vi "NMEA Example - serial.vi"() -> ()   [LabVIEW 2016, in "环境动力监测库.lvlib" / "AIRMAR WeatherCaster.lvlib"]
uses:
  AIRMAR WeatherCaster.lvlib
  NMEA_GPRMC-data.ctl
  NMEA_LatitudeDirection.ctl
  NMEA_LongitudeDirection.ctl
  NMEA_GPVTG-data.ctl
  NMEA_Mode.ctl
  NMEA_GPGGA-data.ctl
  NMEA_GPS-Quality.ctl
  <vilib>/Instr/_visa.llb/VISA Flush IO Buffer Mask.ctl
  <vilib>/Instr/_visa.llb/VISA Configure Serial Port (Instr).vi
panel:
  out "Longitude [deg]":string
  out "Latitude [deg]":string
  in  "time zone":i32
  out "Time":string
  in  "Stop":bool
  in  "VISA":refnum<visa-resource-name>
  in  "Data file path":path
  out "Data":string[][](table)
  out "Raw data GPS":string
  in  "Buffer Size":u32=6400
  in  "Baud rate":u32=115200
  out "TX LAT":dbl
  out "TX LONG":dbl
  out "$GPGGA-message_OUT":T1={"TimeStamp"=timestamp(0 s since 1904-01-01), "Latitude"=0.0, "Latitude-Direction"=enum."", "Longitude"=1.0, "Longitude-Direction"=enum."", "GPS-Quality"=enum."GPS fix (SPS)", "Number of Satellites"=0, "Horizontal Dilution of Precision"=0.0, "Altitude above Mean-Sea-Level"=0.0, "Geoidal separation"=0.0, "Time since last DGPS update"=0.0, "DGPS reference station ID"=0} {"Time since last DGPS update" format="%.02f [s]"; "Geoidal separation" format="%.02f [m]"; "Altitude above Mean-Sea-Level" format="%.02f [m]"; "Horizontal Dilution of Precision" format="%.02f [HDOP]"; "Longitude" format="%0.4f [long]"; "Latitude" format="%.04f [lat]"; "TimeStamp" format="%<%.2X>T"}
  out "$GPVTG-message_OUT":T5={"True Course over Ground"=0.0, "Magnetic Course over Ground"=0.0, "Speed over Ground in knots"=0.0, "Speed over Ground in km/h"=1.0, "Mode"=""} {"Speed over Ground in km/h" format="%.02f [km/h]"; "Speed over Ground in knots" format="%.02f [kts]"; "Magnetic Course over Ground" format="%.02f [deg]"; "True Course over Ground" format="%.02f [deg]"}
  out "$GPRMC-message_OUT":T7={"TimeStamp"=timestamp(0 s since 1904-01-01), "Validity"=FALSE, "Latitude"=0.0, "Latitude-Direction"=enum."North", "Longitude"=0.0, "Longitude-Direction"=enum."East", "Speed in knots"=0.0, "True course"=0.0, "Date Stamp"=timestamp(0 s since 1904-01-01), "Magnetic Variation (East/West)"=0.0} {"Magnetic Variation (East/West)" format="%.02f [deg]"; "Date Stamp" format="%<%x>T"; "True course" format="%.02f [deg]"; "Speed in knots" format="%.02f [kts]"; "Longitude" format="%0.4f [long]"; "Latitude" format="%.04f [lat]"; "TimeStamp" format="%<%.2X>T"}
  # "NMEA EXAMPLE WITH VISA SERIAL"
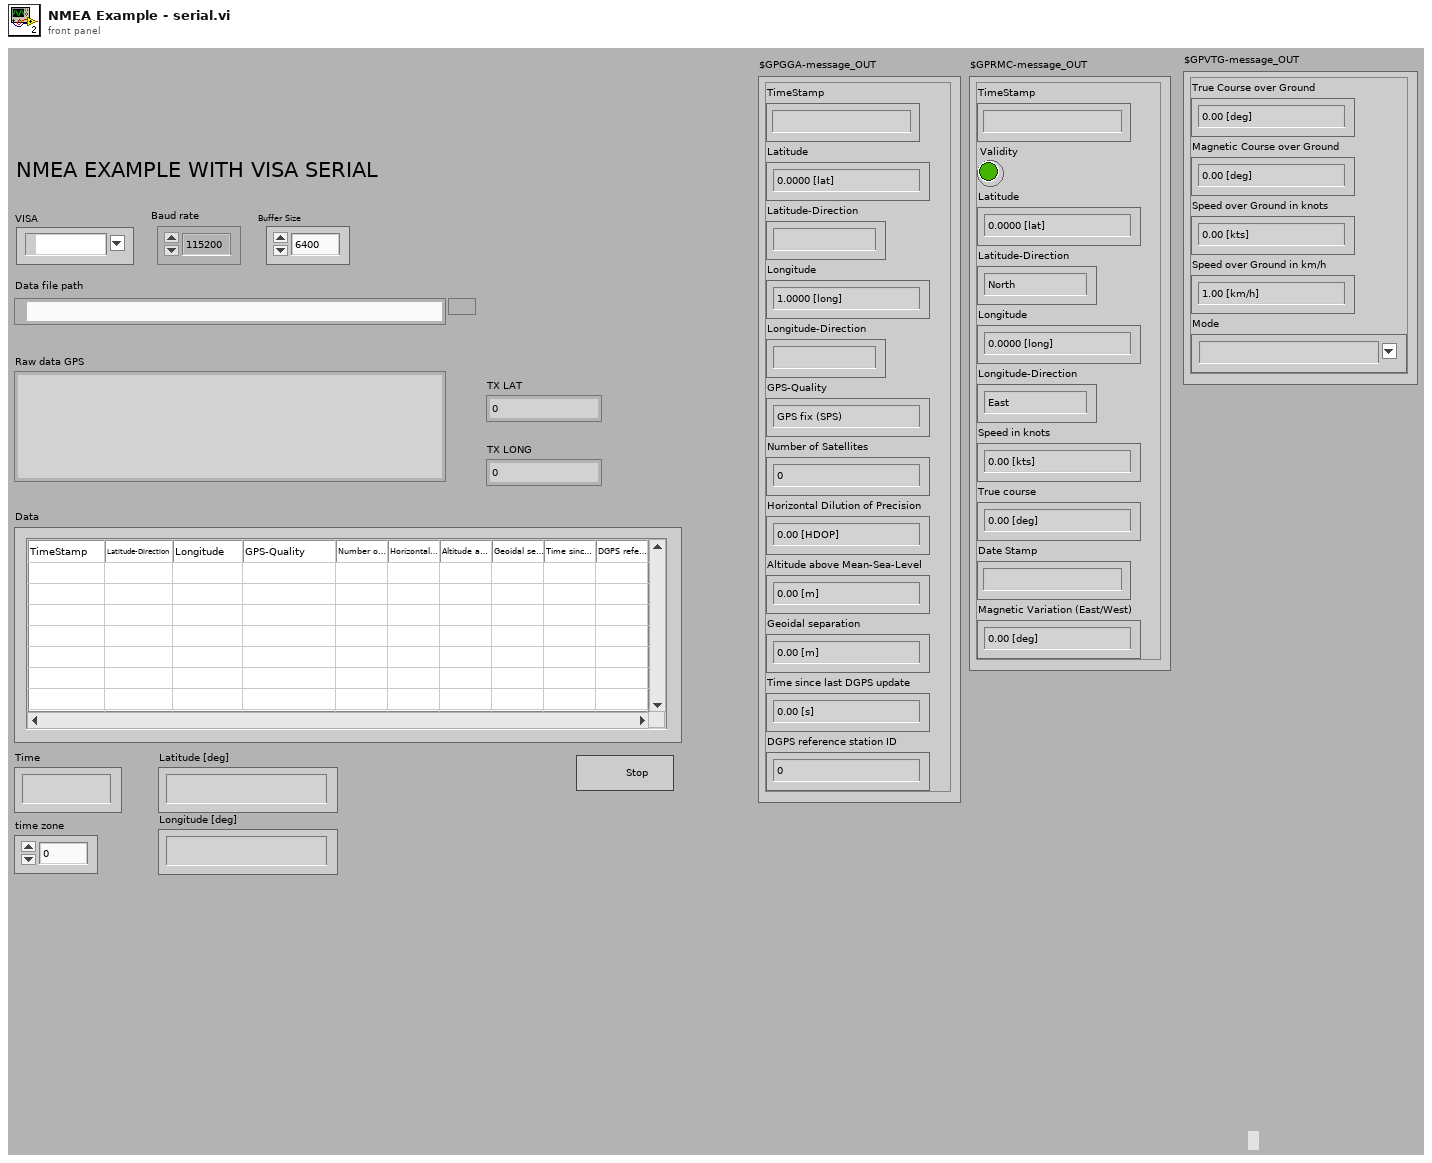
[diagram p1: front panel]
types:
  T1 = typedef "环境动力监测库.lvlib/AIRMAR WeatherCaster.lvlib/NMEA_GPGGA-data.ctl" = cluster{"TimeStamp":timestamp, "Latitude":dbl, "Latitude-Direction":T2, "Longitude":dbl, "Longitude-Direction":T3, "GPS-Quality":T4, "Number of Satellites":i32, "Horizontal Dilution of Precision":dbl, "Altitude above Mean-Sea-Level":dbl, "Geoidal separation":dbl, "Time since last DGPS update":dbl, "DGPS reference station ID":i32}
  T2 = typedef "环境动力监测库.lvlib/AIRMAR WeatherCaster.lvlib/NMEA_LatitudeDirection.ctl" = enum16{"", "North", "South"}
  T3 = typedef "环境动力监测库.lvlib/AIRMAR WeatherCaster.lvlib/NMEA_LongitudeDirection.ctl" = enum16{"", "East", "West"}
  T4 = typedef "环境动力监测库.lvlib/AIRMAR WeatherCaster.lvlib/NMEA_GPS-Quality.ctl" = enum16{"Invalid", "GPS fix (SPS)", "DGPS fix", "PPS fix", "Real Time Kinematic", "Float RTK", "estimated", "Manual input mode", "Simulation mode"}
  T5 = typedef "环境动力监测库.lvlib/AIRMAR WeatherCaster.lvlib/NMEA_GPVTG-data.ctl" = cluster{"True Course over Ground":dbl, "Magnetic Course over Ground":dbl, "Speed over Ground in knots":dbl, "Speed over Ground in km/h":dbl, "Mode":T6}
  T6 = typedef "环境动力监测库.lvlib/AIRMAR WeatherCaster.lvlib/NMEA_Mode.ctl" = string
  T7 = typedef "环境动力监测库.lvlib/AIRMAR WeatherCaster.lvlib/NMEA_GPRMC-data.ctl" = cluster{"TimeStamp":timestamp, "Validity":bool, "Latitude":dbl, "Latitude-Direction":T2, "Longitude":dbl, "Longitude-Direction":T3, "Speed in knots":dbl, "True course":dbl, "Date Stamp":timestamp, "Magnetic Variation (East/West)":dbl}
  T8 = typedef "VISA Flush IO Buffer Mask.ctl" = u16
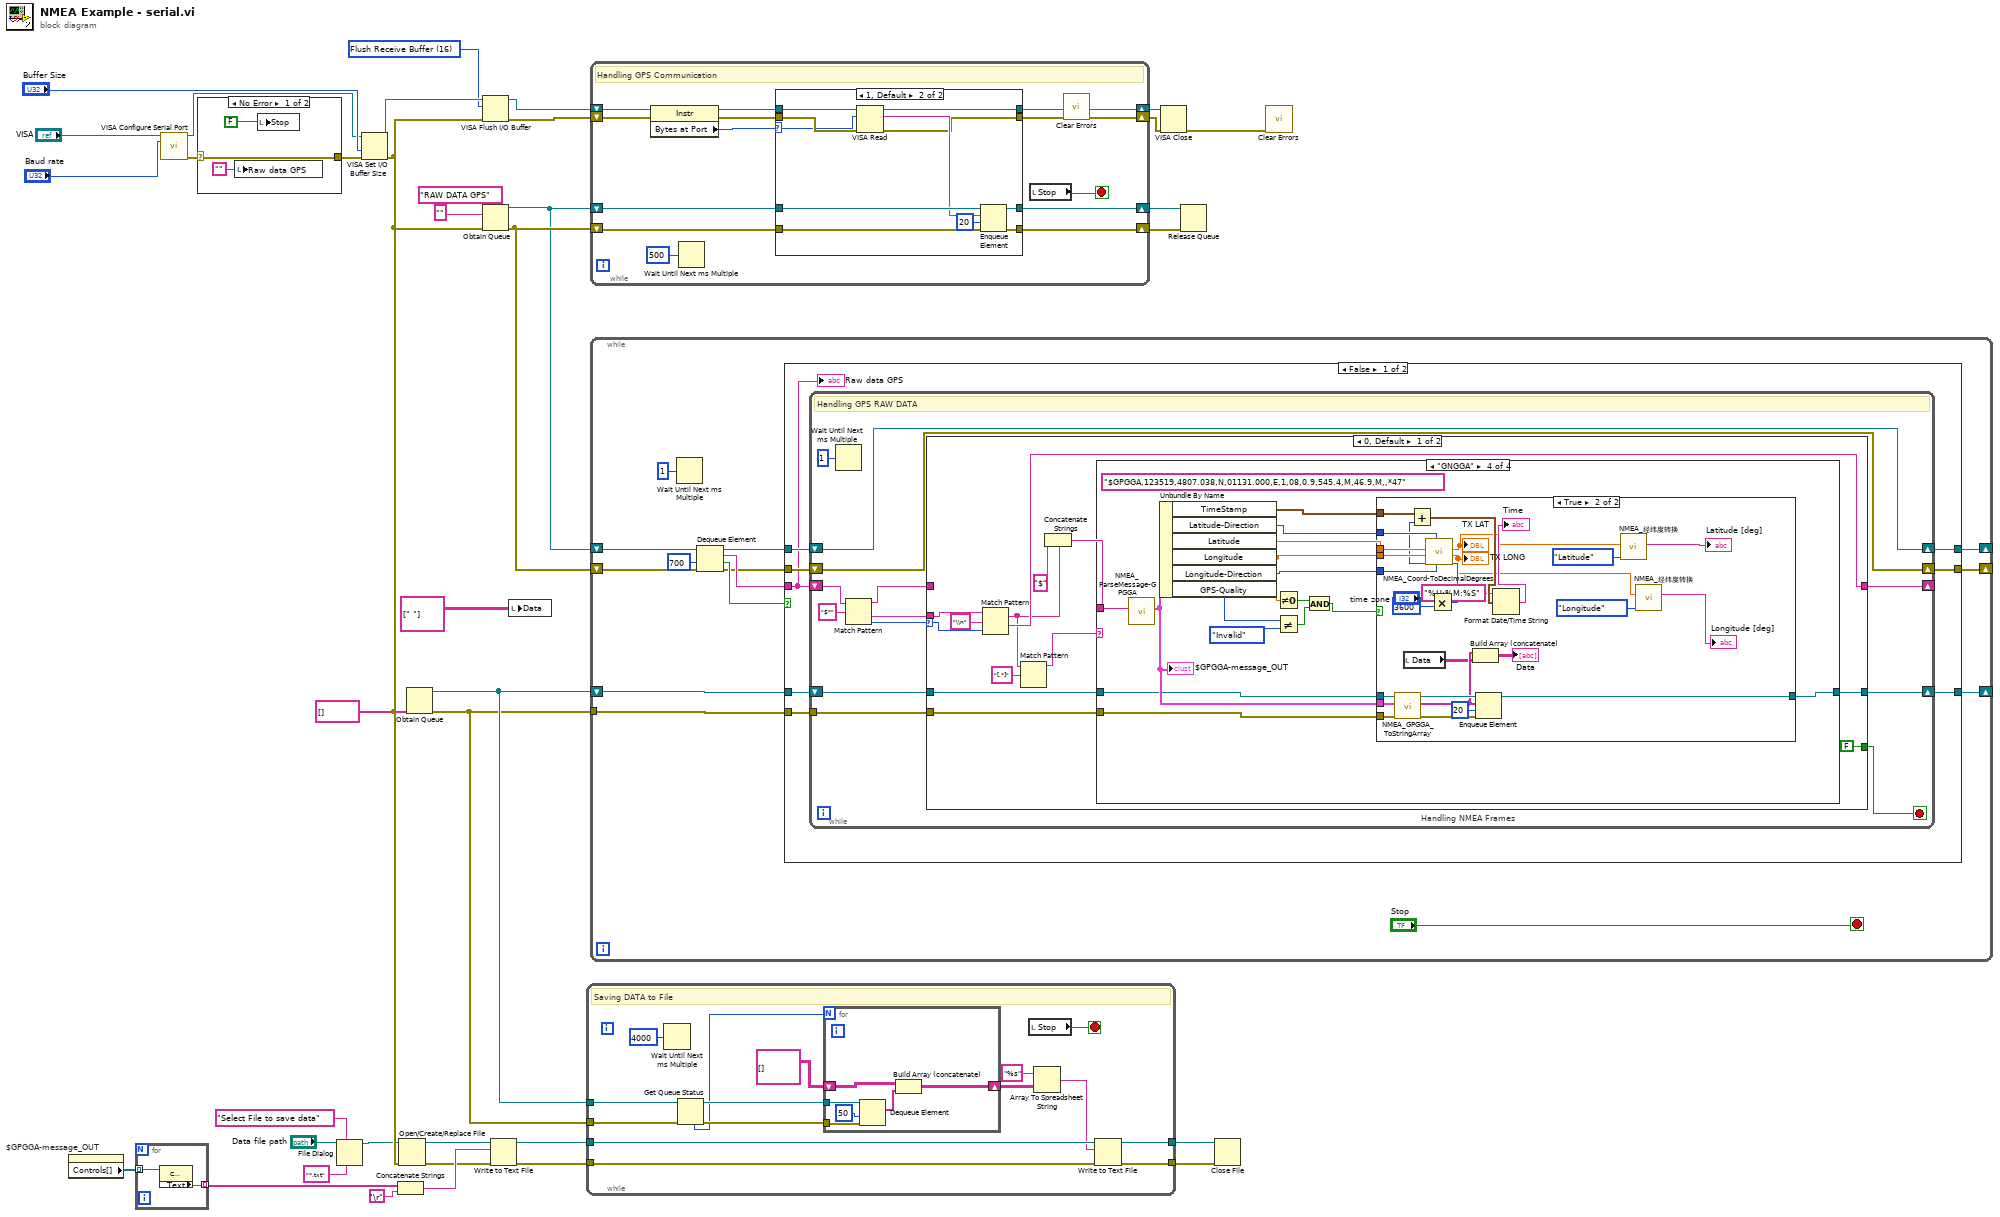
[diagram p0: block diagram]
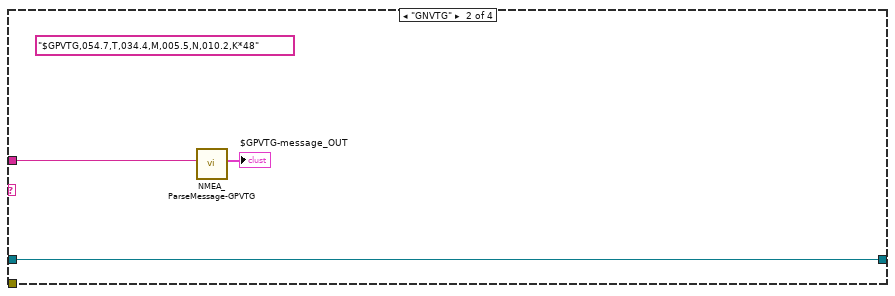
[diagram p5: hidden frame]
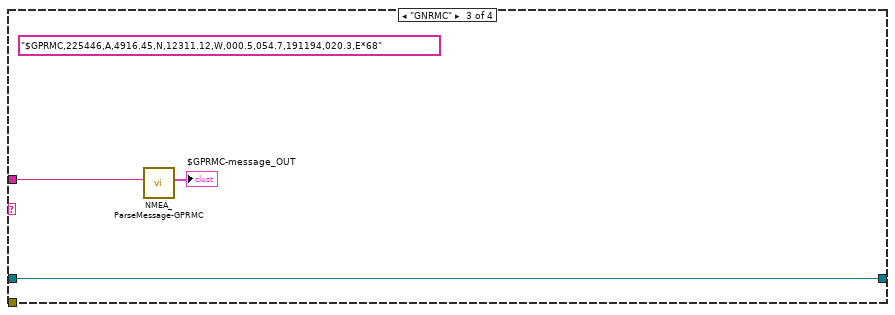
[diagram p6: hidden frame]
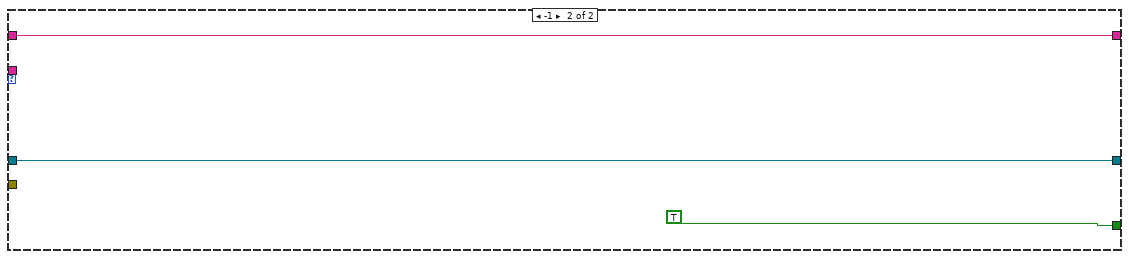
[diagram p8: hidden frame]
diagram:
  w25 = T8 16 items=["Flush Receive Buffer"=16, "Write Transmit Buffer to Device"=32, "Flush Receive Buffer (No I/O)"=64, "Flush Transmit Buffer"=128] ("Mask")
  n1 = property on="$GPGGA-message_OUT" class="Clust (strict)"() -> ("Controls[]"=w13:refnum<vi>[])  [unwired: 2 in, 2 out]
  n2 = for {
    tunnel: w13 -> [w40] mode=indexing
    tunnel: [w39] -> w7 mode=indexing
    n3 = property class="Cmde"(reference=w40) -> ("Label.Text"=w39:string)  [unwired: 1 in, 2 out]
  }
  n4 = call-poly "VISA Configure Serial Port"("VISA resource name"="VISA", "baud rate (9600)"="Baud rate") -> ("VISA resource name out"=w26:refnum<visa-resource-name>, "error out"=w11:errorcluster)  [unwired: 12 in]
  n5 = case shown="No Error" w11 {
    selector: w11 -> [w42 w44]
    tunnel: [w42 w44] -> w9
    frame No Error {
      n6 = local write "Raw data GPS"("") -> ()
      n7 = local write "Stop"(FALSE ("STOP")) -> ()
    }
    frame Error {
    }
  }
  n8 = File Dialog(6:"*.txt" ("filtre (tous les fichiers)"), 7:"Select File to save data" ("message"), 11:"Data file path") -> (3:w3:path)  [unwired: 4 in, 3 out]
  n9 = VISA Set I/O Buffer Size(VISA resource name=w26, size (4096)="Buffer Size", error in (no error)=w9) -> (VISA resource name out=w38:refnum<visa-resource-name>, error out=w8:errorcluster)  [unwired: 1 in]
  n10 = Concatenate Strings(w7, "\r") -> (w32:string)
  n11 = Open/Create/Replace File(file path (use dialog)=w3, error in=w8) -> (refnum out=w16:refnum<file>, error out=w15:errorcluster)  [unwired: 4 in, 1 out]
  n12 = Obtain Queue(element data type=string[] [], error in (no error)=w8) -> (queue out=w31:refnum<queue>, error out=w30:errorcluster)  [unwired: 3 in, 1 out]
  n13 = VISA Flush I/O Buffer(VISA resource name=w38, mask (16)=w25, error in (no error)=w8) -> (VISA resource name out=w37:refnum<visa-resource-name>, error out=w36:errorcluster)
  n14 = Obtain Queue(name (unnamed)="RAW DATA GPS" ("nom (aucun)"), element data type="" ("expression régulière"), error in (no error)=w8) -> (queue out=w21:refnum<queue>, error out=w35:errorcluster)  [unwired: 2 in, 1 out]
  n15 = Write to Text File(file (use dialog)=w16, text=w32, error in=w15) -> (refnum out=w33:refnum<file>, error out=w34:errorcluster)  [unwired: 1 in, 1 out]
  n16 = local write "Data"(string[][] [[" "]]) -> ()
  n17 = while {
    tunnel: [w59] -> w18
    tunnel: [w58] -> w17
    tunnel: w34 -> [w57]
    tunnel: w33 -> [w56]
    tunnel: w31 -> [w50]
    tunnel: w30 -> [w48]
    stop <- w45 stop-if-true
    # "Saving DATA to File"
    n18 = Wait Until Next ms Multiple(millisecond multiple=u32 4000 ("n millisecondes")) -> ()  [unwired: 1 out]
    n19 = Get Queue Status(queue=w50, error in (no error)=w48) -> (queue out=w49:refnum<queue>, error out=w47:errorcluster, # elements in queue=w46:i32)  [unwired: 1 in, 5 out]
    n20 = for {
      N: w46 -> [_]
      shift-right: [w61] -> w54
      shift-left: string[][] [] -> [w65]
      tunnel: w49 -> [w64]
      tunnel: w47 -> [w63]
      n21 = Dequeue Element(queue=w64, timeout in ms (-1)=50 ("timeout en ms (-1)"), error in (no error)=w63) -> (element=w62:string[])  [unwired: 3 out]
      n22 = Build Array (concatenate)(w65, w62) -> (w61:string[][])
    }
    n23 = local read "Stop"() -> (w45:bool)
    n24 = Array To Spreadsheet String(array=w54, 3:"%s" ("format string")) -> (spreadsheet string=w53:string)  [unwired: 1 in]
    n25 = Write to Text File(file (use dialog)=w56, text=w53, error in=w57) -> (refnum out=w59:refnum<file>, error out=w58:errorcluster)  [unwired: 1 in, 1 out]
  }
  n26 = while {
    shift-right: [w76] -> w23
    shift-left: w35 -> [w78]
    shift-right: [w75] -> w20
    shift-left: w37 -> [w74]
    shift-right: [w77] -> w22
    shift-left: w21 -> [w79]
    shift-right: [w67] -> w19
    shift-left: w36 -> [w71]
    stop <- w66 stop-if-true
    # "Handling GPS Communication"
    n27 = property class="Instr"(reference=w74, error in=w71) -> (reference out=w73:refnum<visa-resource-name>, error out=w70:errorcluster, "Bytes at Port"=w68:u32)
    n28 = Wait Until Next ms Multiple(millisecond multiple=u32 500 ("attente (ms)")) -> ()  [unwired: 1 out]
    n29 = case shown="1, Default" w68 {
      selector: w68 -> [_ w85]
      tunnel: w79 -> [w80 w94]
      tunnel: w78 -> [w81 w93]
      tunnel: [w80 w92] -> w77
      tunnel: [w81 w91] -> w76
      tunnel: [w82 w89] -> w75
      tunnel: w73 -> [w82 w88]
      tunnel: w70 -> [w83 w87]
      tunnel: [w83 w86] -> w69
      frame 0 {
      }
      frame 1, Default {
        n30 = VISA Read(VISA resource name=w88, byte count=w85, error in (no error)=w87) -> (VISA resource name out=w89:refnum<visa-resource-name>, read buffer=w90:string, error out=w86:errorcluster)  [unwired: 1 out]
        n31 = Enqueue Element(queue=w94, element=w90, timeout in ms (-1)=20 ("timeout en ms (-1)"), error in (no error)=w93) -> (queue out=w92:refnum<queue>, error out=w91:errorcluster)  [unwired: 1 out]
      }
    }
    n32 = local read "Stop"() -> (w66:bool)
    n33 = call <vilib>:"Clear Errors.vi"("error in (no error)"=w69) -> ("error out"=w67:errorcluster)  [unwired: 5 in, 1 out]
  }
  n34 = while {
    tunnel: w30 -> [w104]
    shift-right: [w102] -> _
    shift-left: w21 -> [w103]
    shift-right: [w98] -> _
    shift-left: w31 -> [w105]
    shift-right: [w97] -> _
    shift-left: w35 -> [w108]
    stop <- "Stop" stop-if-true
    n35 = Wait Until Next ms Multiple(millisecond multiple=u32 1 ("n millisecondes")) -> ()  [unwired: 1 out]
    n36 = Dequeue Element(queue=w103, timeout in ms (-1)=700 ("timeout en ms (-1)"), error in (no error)=w108) -> (queue out=w101:refnum<queue>, element=w107:string, timed out?=w99:bool, error out=w96:errorcluster)
    n37 = case shown="False" w99 {
      tunnel: w107 -> [w109 _]
      tunnel: w105 -> [w116 w195]
      tunnel: w104 -> [w115 _]
      tunnel: [w114 w196] -> w102
      tunnel: w101 -> [w113 w196]
      tunnel: [w112 w195] -> w98
      tunnel: [w111 w194] -> w97
      tunnel: w96 -> [w110 w194]
      frame False {
        n38 = while {
          shift-right: [w127] -> _
          shift-left: w109 -> [w118]
          tunnel: w115 -> [w123]
          shift-right: [w122] -> w114
          shift-left: w113 -> [w122]
          shift-right: [w120] -> w112
          shift-left: w116 -> [w124]
          shift-right: [w119] -> w111
          shift-left: w110 -> [w119]
          stop <- w121 stop-if-true
          # "Handling GPS RAW DATA"
          n39 = Wait Until Next ms Multiple(millisecond multiple=u32 1 ("n millisecondes")) -> ()  [unwired: 1 out]
          n40 = Match Pattern(string=w118, regular expression="$*" ("expression régulière")) -> (before substring=w117:string, after substring=w126:string, offset past match=w128:i32)  [unwired: 1 in, 1 out]
          n41 = case shown="0, Default" w128 {
            selector: w128 -> [w141 _]
            tunnel: [w140 w191] -> w127
            tunnel: w126 -> [w142 _]
            tunnel: [FALSE TRUE] -> w121
            tunnel: w124 -> [w136 w192]
            tunnel: w123 -> [w135 _]
            tunnel: [w133 w192] -> w120
            tunnel: w117 -> [_ w191]
            frame 0, Default {
              n42 = Match Pattern(string=w142, regular expression="\\n" ("expression régulière"), offset (0)=w141) -> (before substring=w132:string, after substring=w140:string)  [unwired: 2 out]
              n43 = Match Pattern(string=w132, regular expression="[,*]" ("正则表达式")) -> (before substring=w130:string)  [unwired: 1 in, 3 out]
              n44 = Concatenate Strings("$" ("expression régulière"), w132) -> (w138:string)
              n45 = case "Handling NMEA Frames" shown="\"GNGGA\"" w130 {
                tunnel: w138 -> [_ w145 w148 w164]
                tunnel: w136 -> [w143 w144 w147 w159]
                tunnel: w135 -> [_ _ _ w158]
                tunnel: [w143 w144 w147 w157] -> w133
                frame " ", Default {
                }
                frame "GNVTG" {
                  (unwired) "$GPVTG,054.7,T,034.4,M,005.5,N,010.2,K*48" ("$GPVTG-message_IN")
                  n46 = call "NMEA_ParseMessage-GPVTG.vi"("$GPVTG-message_IN"=w145) -> ("$GPVTG-message_OUT"=→"$GPVTG-message_OUT":T5)  [unwired: 9 in, 1 out]
                }
                frame "GNRMC" {
                  (unwired) "$GPRMC,225446,A,4916.45,N,12311.12,W,000.5,054.7,191194,020.3,E*68" ("$GPRMC-message_IN")
                  n47 = call "NMEA_ParseMessage-GPRMC.vi"("$GPRMC-message_IN"=w148) -> ("$GPRMC-message_OUT"=→"$GPRMC-message_OUT":T7)  [unwired: 9 in, 1 out]
                }
                frame "GNGGA" {
                  (unwired) "$GPGGA,123519,4807.038,N,01131.000,E,1,08,0.9,545.4,M,46.9,M,,*47" ("data out")
                  n48 = call "NMEA_ParseMessage-GPGGA.vi"("$GPGGA-message_IN"=w164) -> ("$GPGGA-message_OUT"=w160:T1)  [unwired: 9 in, 1 out]
                  "$GPGGA-message_OUT" <- w160
                  n49 = Unbundle By Name(w160) -> ("TimeStamp"=w150:timestamp, "Latitude-Direction"=w161:T2, "Latitude"=w162:dbl, "Longitude"=w156:dbl, "Longitude-Direction"=w163:T3, "GPS-Quality"=w151:T4)
                  n50 = Not Equal To 0?(x=w156) -> (x != 0?=w154:bool)
                  n51 = Not Equal?(x=w151, y=NMEA_GPS-Quality."Invalid" ("GPS-Quality")) -> (x != y?=w152:bool)
                  n52 = Compound Arithmetic op=AND(w154, w152) -> (w155:bool)
                  n53 = case shown="True" w155 {
                    tunnel: w163 -> [_ w190]
                    tunnel: w162 -> [_ w180]
                    tunnel: w161 -> [_ w179]
                    tunnel: w160 -> [_ w189]
                    tunnel: w159 -> [w165 w188]
                    tunnel: w158 -> [_ w187]
                    tunnel: [w165 w183] -> w157
                    tunnel: w156 -> [_ w181]
                    tunnel: w150 -> [_ w178]
                    frame False {
                    }
                    frame True {
                      n54 = call "NMEA_GPGGA_ToStringArray.vi"("$GPGGA-message_IN"=w189) -> ("$GPGGA-message_OUT"=w185:string[])  [unwired: 9 in, 1 out]
                      n55 = local read "Data"() -> (w184:string[][])
                      n56 = call "NMEA_Coord-ToDecimalDegrees.vi"("Longitude-Direction"=w190, "Latitude-Direction"=w179, "Longitude"=w181, "Latitude"=w180) -> ("Longitude"=w167:dbl, "Latitude"=w171:dbl)  [unwired: 6 in]
                      "TX LAT" <- w171
                      "TX LONG" <- w167
                      n57 = Multiply(x="time zone", y=3600) -> (x*y=w175:i32)
                      n58 = Add(x=w178, y=w175) -> (x+y=w174:timestamp)
                      n59 = Build Array (concatenate)(w185, w184) -> (→"Data":string[][])
                      n60 = Enqueue Element(queue=w188, element=w185, timeout in ms (-1)=20 ("timeout en ms (-1)"), error in (no error)=w187) -> (queue out=w183:refnum<queue>)  [unwired: 2 out]
                      n61 = Format Date/Time String(time format string (%c)="%H:%M:%S" ("时间格式字符串(%c)"), seconds (now)=w174) -> (date/time string=→"Time":string)  [unwired: 1 in]
                      n62 = call "NMEA_经纬度转换.vi"("类型"=enum16{"Latitude", "Longitude"}."Latitude", "数值"=w171) -> ("转换结果"=→"Latitude [deg]":string)  [unwired: 9 in]
                      n63 = call "NMEA_经纬度转换.vi"("类型"=enum16{"Latitude", "Longitude"}."Longitude", "数值"=w167) -> ("转换结果"=→"Longitude [deg]":string)  [unwired: 9 in]
                    }
                  }
                }
              }
            }
            frame -1 {
            }
          }
        }
        "Raw data GPS" <- w109
      }
      frame True {
      }
    }
  }
  n64 = VISA Close(VISA resource name=w20, error in (no error)=w19) -> (error out=w24:errorcluster)
  n65 = Release Queue(queue=w22, error in (no error)=w23) -> ()  [unwired: 1 in, 3 out]
  n66 = Close File(refnum=w18, error in=w17) -> ()  [unwired: 2 out]
  n67 = call <vilib>:"Clear Errors.vi"("error in (no error)"=w24) -> ()  [unwired: 5 in, 2 out]
